vi "do_toast.vi"(8 "error in (no error)":errorcluster, 11 "Chef in":refnum<class "Chef.lvclass">) -> (0 "error out":errorcluster, 3 "Chef out":refnum<class "Chef.lvclass">)   [LabVIEW 2020, in "Chef.lvclass"]
uses:
  Chef.lvclass
  Chef.lvclass/Chef.ctl
  Appliance/Appliance.lvclass
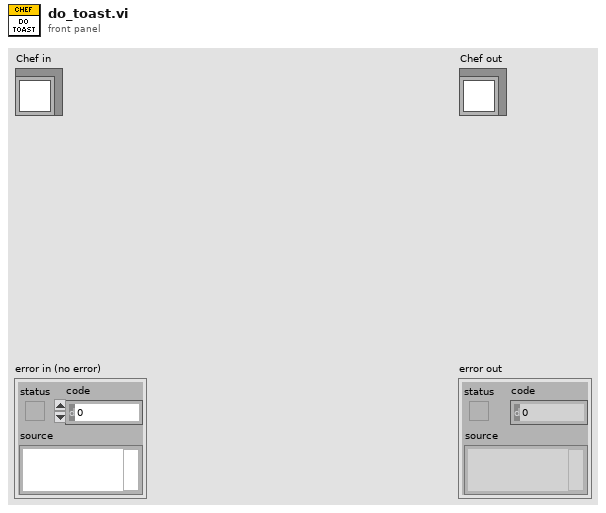
[diagram p1: front panel]
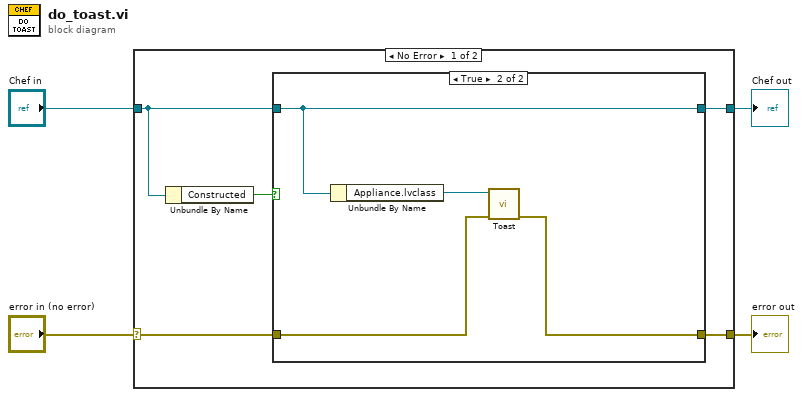
[diagram p0: block diagram]
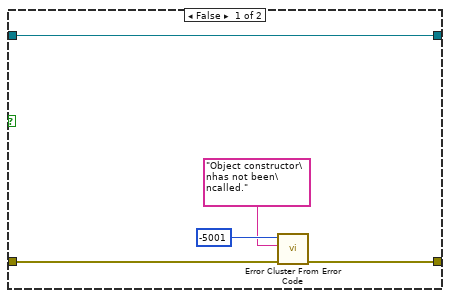
[diagram p2: hidden frame]
diagram:
  n1 = case shown="No Error" "error in (no error)" {
    selector: "error in (no error)" -> [w9 w20]
    tunnel: [w5 w20] -> w3
    tunnel: [w6 w19] -> w1
    tunnel: "Chef in" -> [w7 w19]
    frame No Error {
      n2 = Unbundle By Name(w7) -> ("Constructed"=w8:bool)
      n3 = case shown="True" w8 {
        tunnel: w9 -> [w13 w16]
        tunnel: w7 -> [w14 w18]
        tunnel: [w14 w18] -> w6
        tunnel: [w12 w15] -> w5
        frame False {
          n4 = call <vilib>:"Error Cluster From Error Code.vi"("error in (no error)"=w13, "error message (\"\")"="Object constructor\nhas not been\ncalled." ("error message (\"\")"), "error code (0)"=-5001) -> ("error out"=w12:errorcluster)  [unwired: 6 in]
        }
        frame True {
          n5 = Unbundle By Name(w18) -> ("Appliance.lvclass"=w17:refnum<class "Appliance.lvclass">)
          n6 = call-dynamic "Toast.vi"("error in (no error)"=w16, "Appliance in"=w17) -> ("error out"=w15:errorcluster)  [unwired: 8 in, 1 out]
        }
      }
    }
    frame Error {
    }
  }
  "error out" <- w3
  "Chef out" <- w1
